vi "movement fwd use navX.vi"(8 "error in (no error)":errorcluster) -> (0 "error out":errorcluster)   [LabVIEW 2017]
uses:
  <vilib>/myRIO/Instrument Drivers/Onboard IO/I2C/typedefs/I2C Transfer Rate.ctl
  <vilib>/myRIO/Instrument Drivers/Onboard IO/I2C/I2C.lvlib
  <vilib>/myRIO/Instrument Drivers/Onboard IO/I2C/typedefs/I2C Configuration.ctl
  <vilib>/myRIO/Common/Instrument Driver Framework/myRIO v1.0/I2C/typedefs/I2C Channels Enum.ctl
  <vilib>/myRIO/Common/Instrument Driver Framework/Utilities/typedefs/Generic FPGA Reference.ctl
  <vilib>/myRIO/Common/Instrument Driver Framework/Utilities/typedefs/myRIO v1.0 Reference.ctl
  <vilib>/myRIO/Common/Instrument Driver Framework/Utilities/typedefs/Hardware Version Enum.ctl
  <vilib>/myRIO/Common/Instrument Driver Framework/Utilities/typedefs/myRIO Generic Hardware Reference.ctl
  <vilib>/myRIO/Instrument Drivers/Onboard IO/I2C/typedefs/I2C Reference.ctl
  <vilib>/myRIO/Instrument Drivers/Onboard IO/I2C/vis/myRIO I2C Open.xnode
  <vilib>/myRIO/Instrument Drivers/Utilities/Utilities.lvlib
  <vilib>/myRIO/Common/Instrument Driver Framework/myRIO v1.0/I2C/vis/myRIO v1.1 Open I2C.vi
  <vilib>/userdefined/High Color/nirio_resource_hc.ctl
  <vilib>/imath/engines/lvmath2/RunTimeEngine/Managers/WorkSpace/UID Generator.vi
  <vilib>/imath/engines/lvmath2/RunTimeEngine/LocalVariableDefStatement/MC_LocalVariableDefStatement_Display.vi
  <vilib>/imath/engines/lvmath2/RunTimeEngine/RunTimeType/NIMS_RunTimeType_From StrictType (excl LVString).vi
  <vilib>/imath/engines/lvmath2/RunTimeEngine/VariableToken/NIMS_VariableToken_CondDefined.vi
  <vilib>/imathl/engines/lvmath/Functions/Error Handling/Create Error.vi
  <vilib>/imath/engines/lvmath2/RunTimeEngine/Managers/SymbolTable/Clear UID.vi
  <vilib>/imath/engines/lvmath2/RunTimeEngine/Managers/SymbolTable/NIMS_WorkSpace.lvlib
  <vilib>/imath/engines/lvmath/Functions/Error Handling/MergeErrorsWrapper.vi
  <vilib>/imath/engines/lvmath2/RunTimeEngine/NodeEndStatement/NIMS_NodeEndStatement_Output.vi
  <vilib>/imath/engines/lvmath2/RunTimeEngine/ErrorHandling/NIMS_Finalize Error.vi
panel:
  out "main angle Z":ext
  in  "stop":bool
  out "angle Z":ext
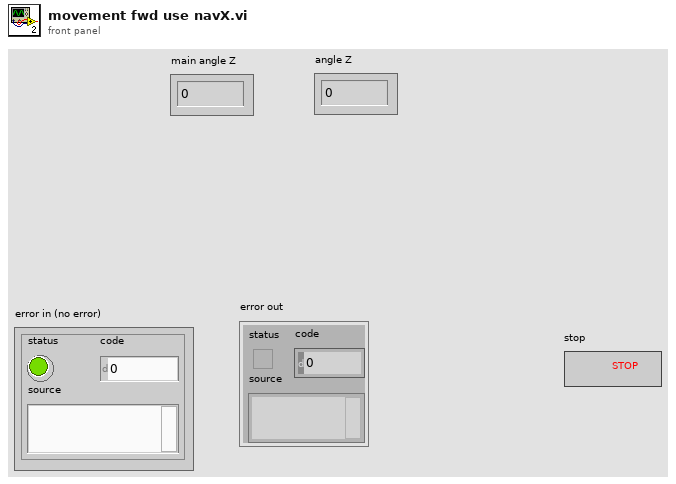
[diagram p1: front panel]
types:
  T1 = typedef "I2C.lvlib/I2C Reference.ctl" = cluster{"myRIO Reference":T2, "I2C Channels Enum":T6, "I2C Configuration":T7}
  T2 = typedef "myRIO Generic Hardware Reference.ctl" = cluster{"myRIO Model":T3, "myRIO Hardware Reference":T4}
  T3 = typedef "Hardware Version Enum.ctl" = enum16{"Unknown", "myRIO-1900", "myRIO-1950", "roboRIO", "NI ELVIS RIO CM"}
  T4 = typedef "myRIO v1.0 Reference.ctl" = cluster{"Generic FPGA Reference":T5, "Allow multiple opens":bool}
  T5 = typedef "Generic FPGA Reference.ctl" = refnum<k20>
  T6 = typedef "I2C Channels Enum.ctl" = enum16{"Not Connected", "A/I2C", "B/I2C", "I2C/I2C"}
  T7 = typedef "I2C.lvlib/I2C Configuration.ctl" = cluster{"I2C Transfer Rate":T8}
  T8 = typedef "I2C.lvlib/I2C Transfer Rate.ctl" = enum16{"Standard mode (100 kbps)", "Fast mode (400 kbps)"}
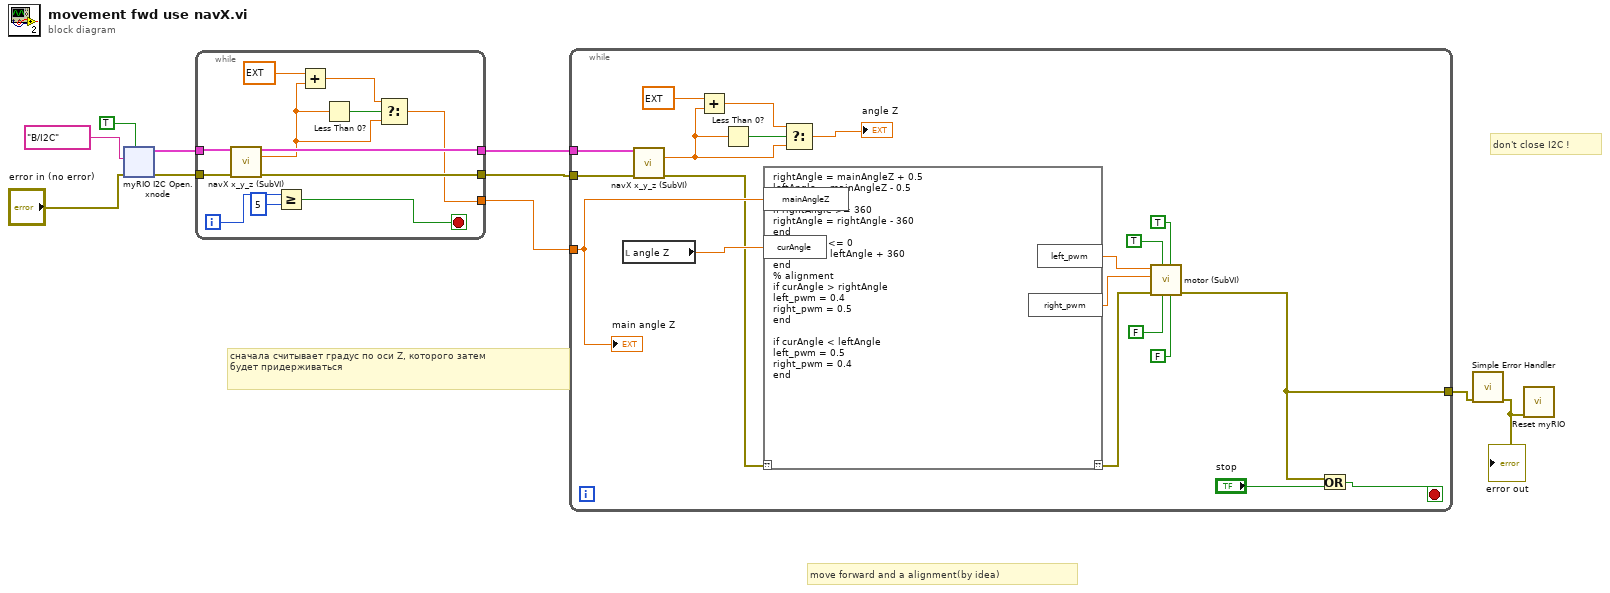
[diagram p0: block diagram]
diagram:
  # "move forward and a alignment(by idea)"
  # "сначала считывает градус по оси Z, которого затем \nбудет придерживаться"
  # "don't close I2C !"
  n1 = xnode "myRIO I2C Open.xnode"("error in (no error)"="error in (no error)", "Allow multiple opens?"=TRUE, "Channel Name"=tag "B/I2C") -> ("error out"=w6:errorcluster, "I2C Ref Out"=w4:T1)
  n2 = while {
    tunnel: [w21] -> w7
    tunnel: w6 -> [w22]
    tunnel: [w13] -> w5
    tunnel: w4 -> [w20]
    tunnel: [w12] -> w3
    i -> [w19]
    stop <- w17 stop-if-true
    n3 = call "navX x_y_z (SubVI).vi"("I2C Ref Out in"=w20, "error in (no error)"=w22) -> ("I2C Ref Out out"=w13:T1, "value Z"=w11:ext, "error out"=w21:errorcluster)  [unwired: 9 in, 2 out]
    n4 = Greater Or Equal?(x=w19, y=5) -> (x >= y?=w17:bool)
    n5 = Add(x=ext 360.0, y=w11) -> (x+y=w15:ext)
    n6 = Less Than 0?(x=w11) -> (x < 0?=w16:bool)
    n7 = Select(t=w15, s=w16, f=w11) -> (s? t:f=w12:ext)
  }
  n8 = while {
    tunnel: w5 -> [w42]
    tunnel: w7 -> [w41]
    tunnel: w3 -> [w35]
    tunnel: [w24] -> w1
    stop <- w23 stop-if-true
    n9 = local read "angle Z"() -> (w34:ext)
    n10 = call "navX x_y_z (SubVI).vi"("I2C Ref Out in"=w42, "error in (no error)"=w41) -> ("value Z"=w36:ext, "error out"=w33:errorcluster)  [unwired: 9 in, 3 out]
    n11 = Add(x=ext 360.0, y=w36) -> (x+y=w38:ext)
    n12 = Less Than 0?(x=w36) -> (x < 0?=w40:bool)
    n13 = mathscript code="rightAngle = mainAngleZ + 0.5\nleftAngle = mainAngleZ - 0.5\n\nif rightAngle >= 360\nrightAngle = rightAngle - 360\nend\nif leftAngle <= 0\nleftAngle = leftAngle + 360\nend\n% alignment\nif curAngle > rightAngle\nleft_pwm = 0.4\nright_pwm = 0.5\nend\n\nif curAngle < leftAngle\nleft_pwm = 0.5\nright_pwm = 0.4\nend"("??"=w33, "mainAngleZ"=w35, "curAngle"=w34) -> ("??"=w28:errorcluster, "right_pwm"=w29:dbl, "left_pwm"=w30:dbl)
    n14 = Select(t=w38, s=w40, f=w36) -> (s? t:f=→"angle Z":ext)
    n15 = call "motor (SubVI).vi"("M1 (Pin 26)"=FALSE, "M1 (Pin 25)"=TRUE, "M0 (Pin 23)"=FALSE, "M0 (Pin 21)"=TRUE, "error in (no error)"=w28, "PWM1"=w29, "PWM0"=w30) -> ("error out"=w24:errorcluster)  [unwired: 4 in]
    n16 = Or(x=w24, y="stop") -> (x .or. y?=w23:bool)
    "main angle Z" <- w35
  }
  n17 = call <vilib>:"Simple Error Handler.vi"("error in (no error)"=w1) -> ("error out"=w2:errorcluster)  [unwired: 4 in, 4 out]
  "error out" <- w2
  n18 = call <vilib>:"Reset myRIO.vi"("error in (no error)"=w2) -> ()  [unwired: 10 in, 1 out]
